vi "0xEC_Read_all_parameters_of_type_float.vi"(8 "error in":errorcluster, 11 "paramUnicorn":T1={"conParam"={"ReadIntParam"=TRUE, "ReadDescrParam"=FALSE, "ReadFloatParam"=TRUE, "debug"=FALSE, "ReadJSON"=TRUE, "IP_address"="192.168.1.216", "N_attempts"=3, "type_con"=enum."TCP", "MB_address"=1, "VISA"="COM1", "connection ID"=refnum, "nameDevices"="", "timeout"=3000, "port"=2000, "type_version"="0F0C0001", "baud_rate"=115200, "VersionControl"=TRUE, "TCP_conn"=TRUE, "WindowSize"=700}, "Param"={"NumParam"={"NTelem"=201, "NInt"=16, "NFloat"=10, "NTable"=2}, "ParamInt"=[{"ID"="Режим работы", "Num"=0, "Name"="", "Type"="", "Enum"="", "Desc"="", "Unit"="", "Access"="", "FormatStr"="", "Min"=0, "Max"=0}, {"ID"="", "Num"=0, "Name"="", "Type"="", "Enum"="", "Desc"="", "Unit"="", "Access"="", "FormatStr"="", "Min"=0, "Max"=0}, {"ID"="", "Num"=0, "Name"="", "Type"="", "Enum"="", "Desc"="", "Unit"="", "Access"="", "FormatStr"="", "Min"=0, "Max"=0}, {"ID"="", "Num"=0, "Name"="", "Type"="", "Enum"="", "Desc"="", "Unit"="", "Access"="", "FormatStr"="", "Min"=0, "Max"=0}, {"ID"="", "Num"=0, "Name"="", "Type"="", "Enum"="", "Desc"="", "Unit"="", "Access"="", "FormatStr"="", "Min"=0, "Max"=0}, {"ID"="", "Num"=0, "Name"="", "Type"="", "Enum"="", "Desc"="", "Unit"="", "Access"="", "FormatStr"="", "Min"=0, "Max"=0}, {"ID"="ModeWork", "Num"=0, "Name"="", "Type"="", "Enum"="", "Desc"="", "Unit"="", "Access"="", "FormatStr"="", "Min"=0, "Max"=0}], "Telemetry"=[], "Table"=[], "ParamFloat"=[]}}) -> (0 "error out":errorcluster, 1 "ArrayFloatStr":string[][](array[string]), 2 "ArrayFloat":sgl[](array[numeric]), 3 "paramUnicorn 2":T1={"conParam"={"ReadIntParam"=TRUE, "ReadDescrParam"=FALSE, "ReadFloatParam"=TRUE, "debug"=FALSE, "ReadJSON"=TRUE, "IP_address"="192.168.1.216", "N_attempts"=3, "type_con"=enum."TCP", "MB_address"=1, "VISA"="COM1", "connection ID"=refnum, "nameDevices"="", "timeout"=3000, "port"=2000, "type_version"="0F0C0001", "baud_rate"=115200, "VersionControl"=TRUE, "TCP_conn"=TRUE, "WindowSize"=700}, "Param"={"NumParam"={"NTelem"=201, "NInt"=16, "NFloat"=10, "NTable"=2}, "ParamInt"=[{"ID"="Режим работы", "Num"=0, "Name"="", "Type"="", "Enum"="", "Desc"="", "Unit"="", "Access"="", "FormatStr"="", "Min"=0, "Max"=0}, {"ID"="", "Num"=0, "Name"="", "Type"="", "Enum"="", "Desc"="", "Unit"="", "Access"="", "FormatStr"="", "Min"=0, "Max"=0}, {"ID"="", "Num"=0, "Name"="", "Type"="", "Enum"="", "Desc"="", "Unit"="", "Access"="", "FormatStr"="", "Min"=0, "Max"=0}, {"ID"="", "Num"=0, "Name"="", "Type"="", "Enum"="", "Desc"="", "Unit"="", "Access"="", "FormatStr"="", "Min"=0, "Max"=0}, {"ID"="", "Num"=0, "Name"="", "Type"="", "Enum"="", "Desc"="", "Unit"="", "Access"="", "FormatStr"="", "Min"=0, "Max"=0}, {"ID"="", "Num"=0, "Name"="", "Type"="", "Enum"="", "Desc"="", "Unit"="", "Access"="", "FormatStr"="", "Min"=0, "Max"=0}, {"ID"="ModeWork", "Num"=0, "Name"="", "Type"="", "Enum"="", "Desc"="", "Unit"="", "Access"="", "FormatStr"="", "Min"=0, "Max"=0}], "Telemetry"=[], "Table"=[], "ParamFloat"=[]}})   [LabVIEW 2017, in "LV_Unicorn.lvlib"]
uses:
  LV_Unicorn.lvlib
  Control/unicorn_Param.ctl
  Control/unicorn_conn.ctl
  Control/unicorn_JSON.ctl
  Control/unicorn_ParamInt.ctl
  Control/unicorn_Telemetry.ctl
  Control/unicorn_Table.ctl
  Control/unicorn_ParamFloat.ctl
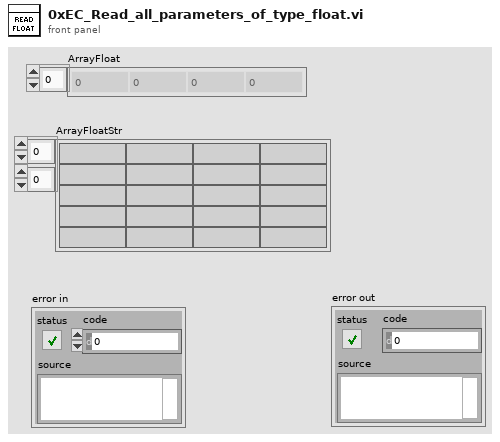
[diagram p1: front panel]
types:
  T1 = typedef "LV_Unicorn.lvlib/unicorn_Param.ctl" = cluster{"conParam":T2, "Param":T3}
  T2 = typedef "LV_Unicorn.lvlib/unicorn_conn.ctl" = cluster{"ReadIntParam":bool, "ReadDescrParam":bool, "ReadFloatParam":bool, "debug":bool, "ReadJSON":bool, "IP_address":string, "N_attempts":i32, "type_con":enum16{"Serial", "TCP"}, "MB_address":i32, "VISA":refnum<visa-resource-name>, "connection ID":refnum<k5>, "nameDevices":string, "timeout":i32, "port":u16, "type_version":string, "baud_rate":u32, "VersionControl":bool, "TCP_conn":bool, "WindowSize":i32}
  T3 = typedef "LV_Unicorn.lvlib/unicorn_JSON.ctl" = cluster{"NumParam":cluster{"NTelem":i32, "NInt":i32, "NFloat":i32, "NTable":i32}, "ParamInt":T4, "Telemetry":T5, "Table":T6, "ParamFloat":T7}
  T4 = typedef "LV_Unicorn.lvlib/unicorn_ParamInt.ctl" = cluster{"ID":string, "Num":i32, "Name":string, "Type":string, "Enum":string, "Desc":string, "Unit":string, "Access":string, "FormatStr":string, "Min":i32, "Max":i32}[]
  T5 = typedef "LV_Unicorn.lvlib/unicorn_Telemetry.ctl" = cluster{"ID":string, "Num":i32, "Name":string, "Desc":string, "Unit":string, "FormatStr":string, "Min":i32, "Max":i32}[]
  T6 = typedef "LV_Unicorn.lvlib/unicorn_Table.ctl" = cluster{"Num":i32, "Access":string, "ColumnCount":i32, "NeedParamPrepare":bool, "Columns":cluster{"Column":i32, "Desc":string, "Name":string}[], "DataType":string, "FormatStr":string, "ID":string, "Name":string, "RowCount":i32, "Rows":cluster{"Desc":string, "ID":string, "Max":i32, "Min":i32, "Name":string, "Row":i32, "Unit":string}[], "Type":string}[]
  T7 = typedef "LV_Unicorn.lvlib/unicorn_ParamFloat.ctl" = cluster{"ID":string, "Num":i32, "Name":string, "Type":string, "Enum":string, "Desc":string, "Unit":string, "Access":string, "FormatStr":string, "Min":sgl, "Max":sgl}[]
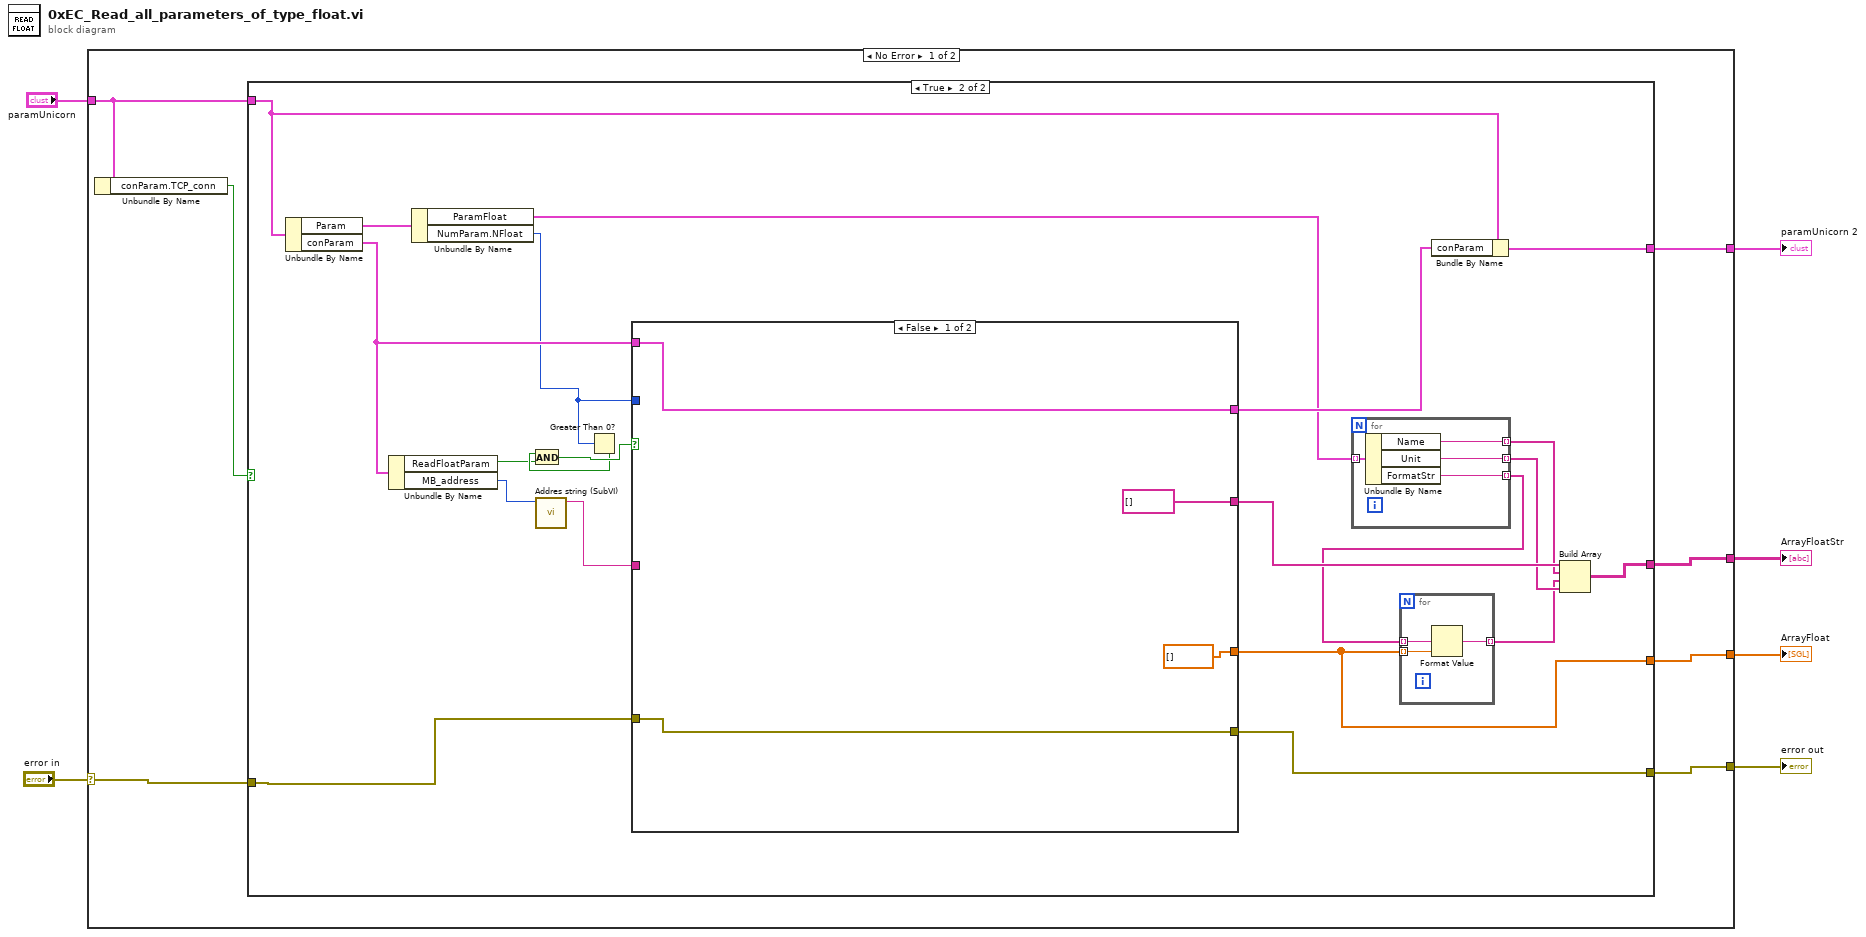
[diagram p0: block diagram]
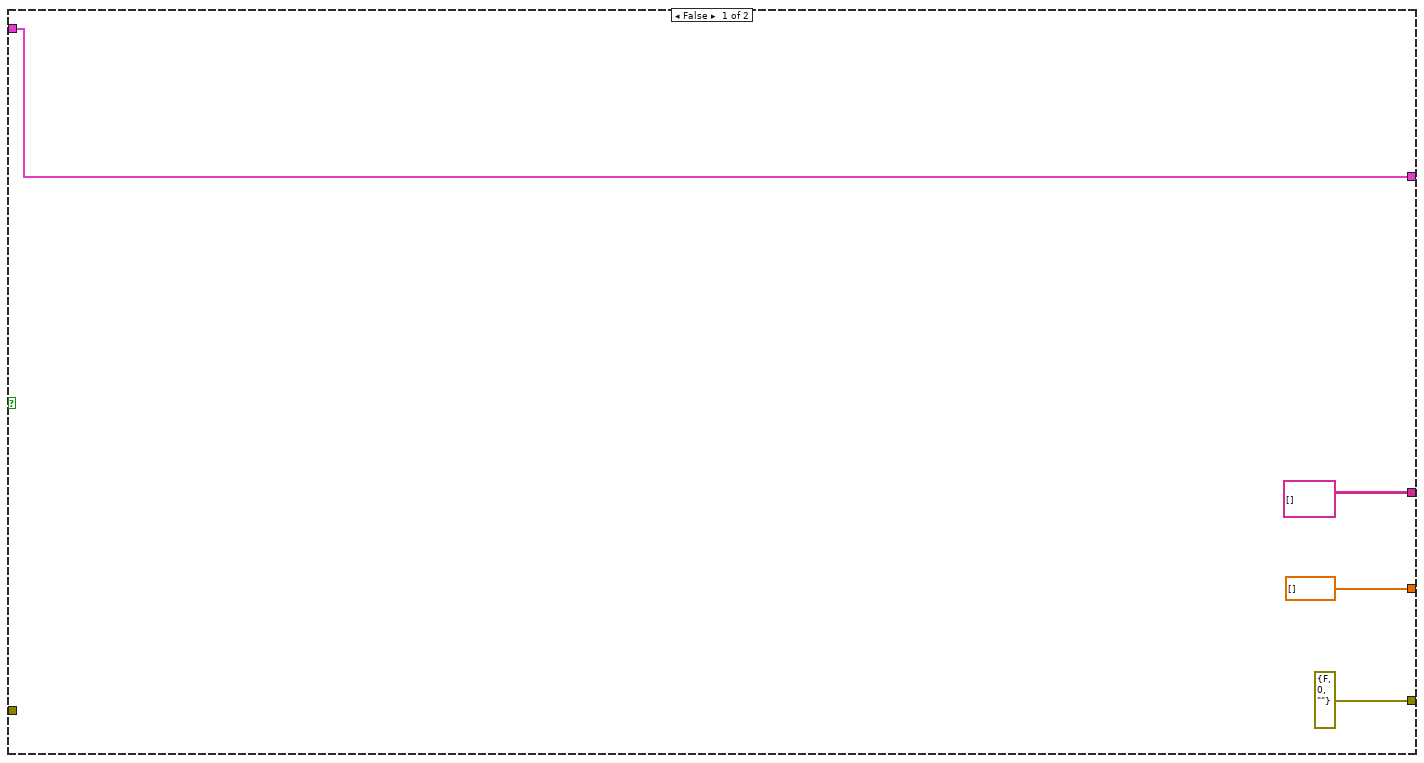
[diagram p2: hidden frame]
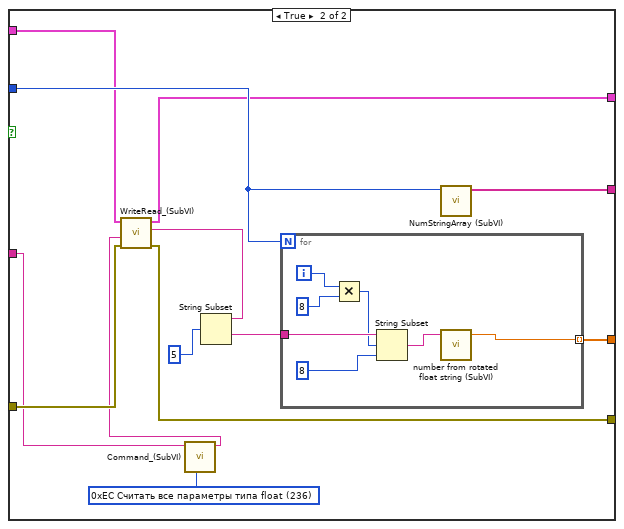
[diagram p3: hidden frame]
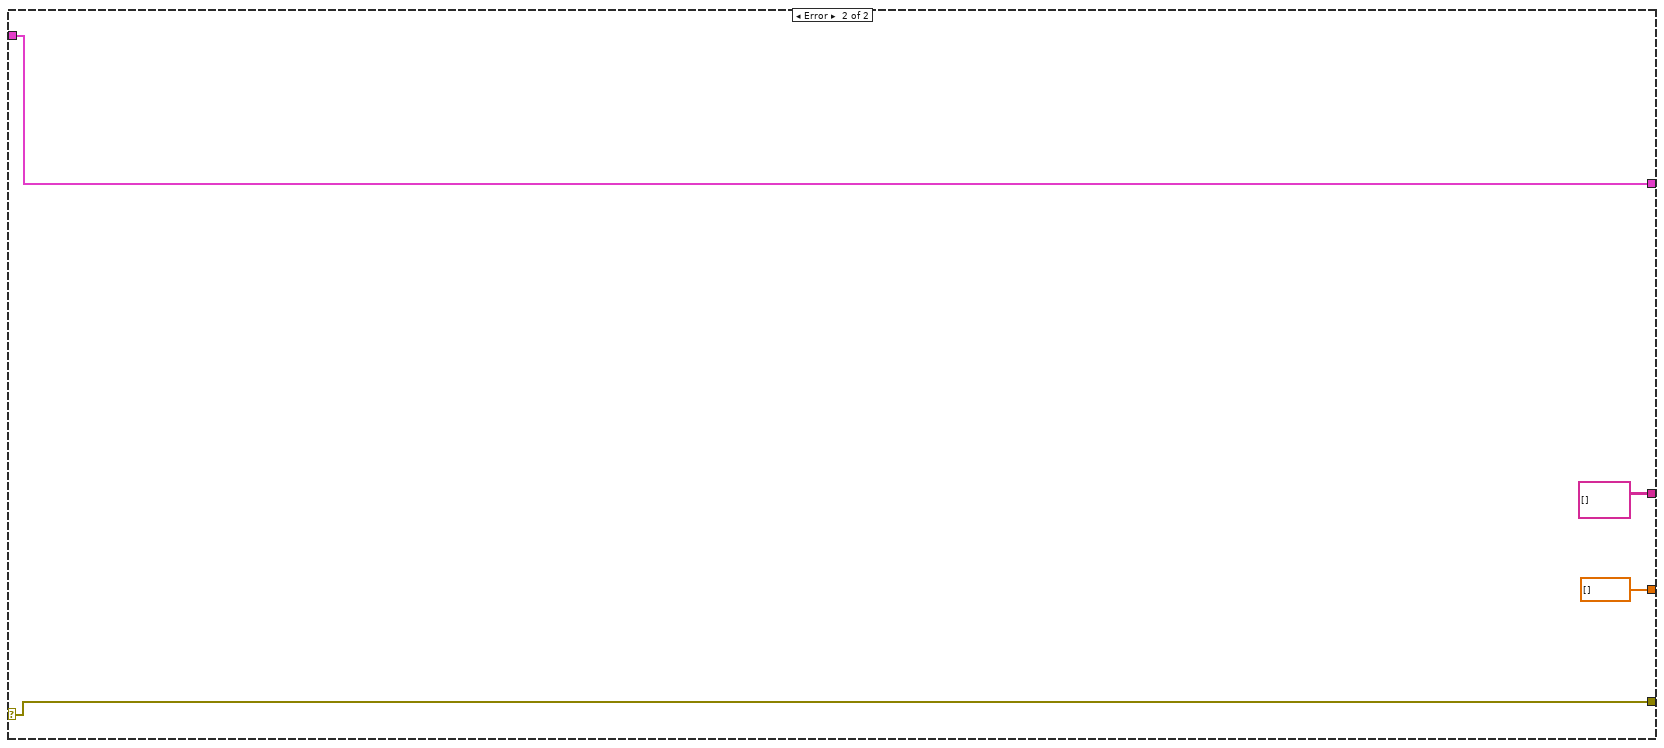
[diagram p4: hidden frame]
diagram:
  n1 = case shown="No Error" "error in" {
    selector: "error in" -> [w9 w70]
    tunnel: [w13 w70] -> w6
    tunnel: [w12 string[][] []] -> w5
    tunnel: [w11 sgl[] []] -> w4
    tunnel: "paramUnicorn" -> [w8 w73]
    tunnel: [w10 w73] -> w2
    frame No Error {
      n2 = Unbundle By Name(w8) -> ("conParam.TCP_conn"=w7:bool)
      n3 = case shown="True" w7 {
        tunnel: [errorcluster {"status"=FALSE, "code"=0, "source"=""} ("error out") w38] -> w13
        tunnel: [string[][] [] w37] -> w12
        tunnel: [sgl[] [] w18] -> w11
        tunnel: w8 -> [w17 w34]
        tunnel: [w17 w32] -> w10
        tunnel: w9 -> [_ w24]
        frame False {
        }
        frame True {
          n4 = Unbundle By Name(w34) -> ("Param"=w35:T3, "conParam"=w36:T2)
          n5 = Unbundle By Name(w36) -> ("ReadFloatParam"=w26:bool, "MB_address"=w31:i32)
          n6 = Unbundle By Name(w35) -> ("ParamFloat"=w23:T7, "NumParam.NFloat"=w25:i32)
          n7 = call "Addres string (SubVI).vi"("Адрес"=w31) -> ("String"=w30:string)  [unwired: 10 in]
          n8 = Greater Than 0?(x=w25) -> (x > 0?=w27:bool)
          n9 = And(x=w27, y=w26) -> (x .and. y?=w28:bool)
          n10 = case shown="False" w28 {
            tunnel: w25 -> [_ w59]
            tunnel: [string[] [] ("Array") w58] -> w29
            tunnel: w30 -> [_ w51]
            tunnel: w36 -> [w47 w57]
            tunnel: w24 -> [w48 w56]
            tunnel: [w48 w55] -> w38
            tunnel: [w47 w54] -> w33
            tunnel: [sgl[] [] w53] -> w18
            frame False {
            }
            frame True {
              w52 = u16 236 items=["0xE0 Запрос количества доступных параметров"=224, "0xE1 Записать один параметр типа float"=225, "0xE2 Записать один параметр типа int"=226, "0xE3 Считать один параметр телеметрии"=227, "0xE4 Записать все параметры типа float"=228, "0xE5 Записать все параметры типа int"=229, "0xE6 Считать все данные телеметрии"=230, "0xE7 Получить описание одного параметра типа float"=231, "0xE8 Получить описание одного параметра типа int"=232, "0xE9 Получить описание одного параметра телеметрии"=233, "0xEA Считать один параметр типа float"=234, "0xEB Считать один параметр типа int"=235, "0xEC Считать все параметры типа float"=236, "0xED Считать все параметры типа int"=237, "0xEE Считать считать фрагмент описания устройства в формате JSON"=238, "0x06 Записать UUID"=6, "0x07 Чтение UUID"=7, "0x45 Считывание параметров Flash памяти"=69, "0x43 Запись страницы Flash памяти"=67, "0x44 Чтения страницы Flash памяти"=68, "0x46 Получить описание Flash-памяти"=70, "0xFA Программный сброс"=250, "0xFB Изменение скорости интерфейса"=251, "0xFF Считывание типа и версии устройства"=255, "0x50 Запрос кол-ва табличных параметров"=80, "0x51 Запрос описания табличного параметра"=81, "0x52 Чтение данных табличного параметра"=82, "0x53 Запись данных табличного параметра"=83, "0x54 Подготовка табличного параметра"=84, "0x55 Запрос прогресса подготовки табличного параметра"=85, "0x56 Освобождение данных подготовленного табличного параметра"=86] ("Команда")
              n11 = call "Command_(SubVI).vi"("Команда"=w52, "String in"=w51) -> ("String out"=w50:string)  [unwired: 9 in]
              n12 = call "WriteRead_(SubVI).vi"("error in"=w56, "Запрос"=w50, "ParamIn"=w57) -> ("error out"=w55:errorcluster, "Ответ"=w60:string, "ParamOut"=w54:T2)  [unwired: 4 in, 2 out]
              n13 = String Subset(string=w60, offset (0)=5) -> (substring=w61:string)  [unwired: 1 in]
              n14 = for {
                N: w59 -> [_]
                tunnel: w61 -> [w69]
                tunnel: [w63] -> w53 mode=indexing
                i -> [w66]
                n15 = Multiply(x=w66, y=i8 8) -> (x*y=w65:i32)
                n16 = String Subset(string=w69, offset (0)=w65, length (rest)=8 ("length (rest)")) -> (substring=w64:string)
                n17 = call "number from rotated float string (SubVI).vi"("String"=w64) -> ("rotated float number"=w63:sgl)  [unwired: 2 in, 2 out]
              }
              n18 = call "NumStringArray (SubVI).vi"("NInt"=w59) -> ("Array"=w58:string[])  [unwired: 10 in]
            }
          }
          n19 = for {
            tunnel: w23 -> [w45] mode=indexing
            tunnel: [w44] -> w22 mode=indexing
            tunnel: [w43] -> w21 mode=indexing
            tunnel: [w42] -> w20 mode=indexing
            n20 = Unbundle By Name(w45) -> ("Name"=w44:string, "Unit"=w43:string, "FormatStr"=w42:string)
          }
          n21 = for {
            tunnel: w18 -> [w41] mode=indexing
            tunnel: w20 -> [w40] mode=indexing
            tunnel: [w39] -> w19 mode=indexing
            n22 = Format Value(format string=w40, value (0)=w41) -> (output string=w39:string)  [unwired: 1 in]
          }
          n23 = Bundle By Name(cluster=w34, "conParam"=w33) -> (w32:T1)
          n24 = Build Array(w29, w22, w19, w21) -> (w37:string[][])
        }
      }
    }
    frame Error {
    }
  }
  "error out" <- w6
  "ArrayFloatStr" <- w5
  "ArrayFloat" <- w4
  "paramUnicorn 2" <- w2
